vi "振动判定.vi"(7 "Result":refnum<vi>, 9 "振动判定":T1, 10 "振动判定范围":T2, 11 "FFT":cluster{"f0":dbl, "df":dbl, "magnitude":dbl[]}[](graph)) -> (2 "FFT 2":cluster{"f0":dbl, "df":dbl, "magnitude":dbl[]}[](graph), 3 "OK？":bool)   [LabVIEW 2020]
uses:
  Global_Variable/Global1.vi
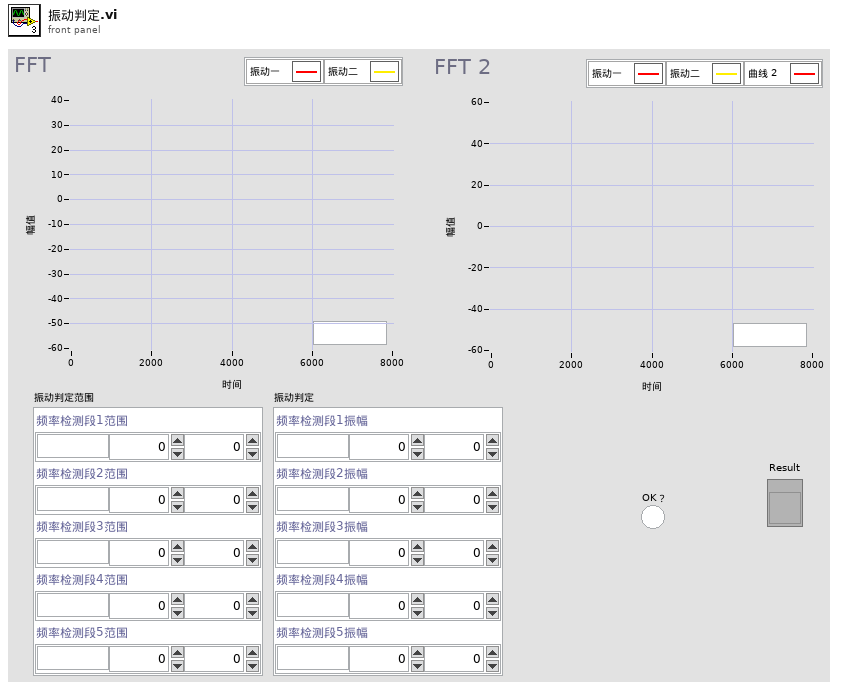
[diagram p1: front panel]
types:
  T1 = cluster{"频率检测段1振幅":cluster{"单位":string, "下限":dbl, "上限":dbl}, "频率检测段2振幅":cluster{"单位":string, "下限":dbl, "上限":dbl}, "频率检测段3振幅":cluster{"单位":string, "下限":dbl, "上限":dbl}, "频率检测段4振幅":cluster{"单位":string, "下限":dbl, "上限":dbl}, "频率检测段5振幅":cluster{"单位":string, "下限":dbl, "上限":dbl}}
  T2 = cluster{"频率检测段1范围":cluster{"单位":string, "下限":dbl, "上限":dbl}, "频率检测段2范围":cluster{"单位":string, "下限":dbl, "上限":dbl}, "频率检测段3范围":cluster{"单位":string, "下限":dbl, "上限":dbl}, "频率检测段4范围":cluster{"单位":string, "下限":dbl, "上限":dbl}, "频率检测段5范围":cluster{"单位":string, "下限":dbl, "上限":dbl}}
  T3 = typedef "svc_Spectrum Info.ctl" = cluster{"channel name":string, "description":string, "x-axis units":T4, "spectral info":cluster{"spectrum type":T5, "linear/dB":enum16{"linear", "dB"}, "window":u16, "window size":i32, "FFT size":i32}, "engineering units":T6, "custom label":string, "dB reference [EU]":dbl, "peak units":enum16{"rms", "peak", "peak-peak"}, "weighting filter":T7, "spectral density?":bool, "unit label":string, "spectrum skewed?":bool, "complimentary spectrum units":T8}
  T4 = typedef "svc_X-Axis Units.ctl" = u16
  T5 = typedef "svc_Spectrum Type.ctl" = enum16{"FFT Spectrum [complex]", "Amplitude [Magnitude]", "Power [Magnitude^2]", "Cross Spectrum [complex]", "Frequency Response [Complex]"}
  T6 = typedef "svc_Engineering Units Text Ring.ctl" = u16
  T7 = typedef "svc_Weighting Filter Text Ring.ctl" = u16
  T8 = typedef "svc_Complimentary Spectrum Units.ctl" = enum16{"none", "radians", "degrees", "cycles", "imaginary"}
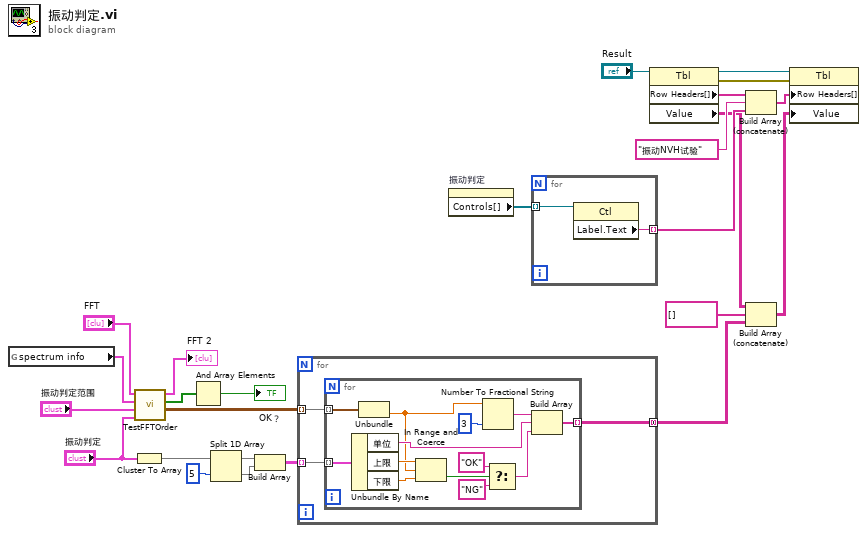
[diagram p0: block diagram]
diagram:
  n1 = global read "Global1.vi" "spectrum info"() -> (w24:T3[])
  n2 = Cluster To Array(cluster="振动判定") -> (array=w8:cluster{"单位":string, "下限":dbl, "上限":dbl}[])
  n3 = call "TestFFTOrder.vi"("振动判定"="振动判定", "振动判定范围"="振动判定范围", "spectrum info"=w24, "FFT 5"="FFT") -> ("数组"=w14:cluster{"freq.":dbl, "dB":dbl}[][], "Test Result"=w1:bool[], "FFT 2"=→"FFT 2":cluster{"x0":dbl, "dx":dbl, "Y":dbl[]}[])  [unwired: 5 in]
  n4 = And Array Elements(Boolean array=w1) -> (logical AND=→"OK？":bool)
  n5 = Split 1D Array(array=w8, index=5 ("索引")) -> (first subarray=w7:cluster{"单位":string, "下限":dbl, "上限":dbl}[], second subarray=w6:cluster{"单位":string, "下限":dbl, "上限":dbl}[])
  n6 = Build Array(w7, w6) -> (w5:cluster{"单位":string, "下限":dbl, "上限":dbl}[][])
  n7 = for {
    tunnel: w14 -> [w28] mode=indexing
    tunnel: [w26] -> w3 mode=concatenating
    tunnel: w5 -> [w27] mode=indexing
    n8 = for {
      tunnel: w28 -> [w41] mode=indexing
      tunnel: w27 -> [w39] mode=indexing
      tunnel: [w34] -> w26 mode=indexing
      n9 = Unbundle By Name(w39) -> ("单位"=w36:string, "上限"=w31:dbl, "下限"=w32:dbl)
      n10 = Unbundle(w41) -> ("dB"=w30:dbl)  [unwired: 1 out]
      n11 = In Range and Coerce(upper limit=w31, x=w30, lower limit=w32) -> (In Range?=w29:bool)  [unwired: 1 out]
      n12 = Number To Fractional String(number=w30, precision (6)=i16 3 ("精度(6)")) -> (F-format string=w35:string)  [unwired: 2 in]
      n13 = Select(t="OK", s=w29, f="NG") -> (s? t:f=w37:string)
      n14 = Build Array(w35, w36, w37) -> (w34:string[])
    }
  }
  n15 = property on="振动判定" class="Clust (严格)"() -> ("Controls[]"=w16:refnum<vi>[])  [unwired: 2 in, 2 out]
  n16 = for {
    tunnel: w16 -> [w43] mode=indexing
    tunnel: [w42] -> w15 mode=indexing
    n17 = property class="Ctl"(reference=w43) -> ("Label.Text"=w42:string)  [unwired: 1 in, 2 out]
  }
  n18 = property class="Tbl"(reference="Result") -> (reference out=w21:refnum<vi>, error out=w22:errorcluster, "Row Headers[]"=w18:string[], "Value"=w13:string[][])  [unwired: 1 in]
  n19 = Build Array (concatenate)(w18, "振动NVH试验" ("Label.Text"), w15) -> (w20:string[])
  n20 = Build Array (concatenate)(w13, string[] [] ("Label.Text"), w3) -> (w12:string[][])
  n21 = property class="Tbl"(reference=w21, error in=w22, "Row Headers[]"=w20, "Value"=w12) -> ()  [unwired: 2 out]
